vi "SDCP SMF Receiver and Trasmitter - Live Plot.vi"() -> ()   [LabVIEW 2020]
uses:
  Typedefs/SDCP - Standard Message Frame Parameters - FGV - commands.ctl
  Typedefs/SDCP - Serial Port Control - Commands.ctl
  Global Stop.vi
panel:
  in  "SYNC":bool
  out "Update to loop":bool
  out "Ranges to loop":T1(array[cluster])
  out "All offsets":dbl[](array[numeric])
  in  "Offset (%)":dbl
  out "Ranges":T1(array[cluster])
  in  "Set range":bool
  in  "Get range":bool
  in  "Auto range":bool
  in  "Maximum":dbl
  in  "Minimum":dbl
  out "Active Plot Names":string[](array[string])
  out "Value":dbl
  out "Time (ms)":dbl
  in  "Current Parameter":string(combo)
  out "Instantaeneous data":T2(array[cluster])
  in  "Time span (ms)":dbl=20000.0
  in  "Channel 8 enable":bool
  in  "Channel 7 enable":bool
  in  "Channel 6 enable":bool
  in  "Channel 5 enable":bool
  in  "Channel 4 enable":bool
  in  "Channel 3 enable":bool
  in  "Channel 2 enable":bool
  in  "Channel 1 enable":bool
  in  "Channel 8 parameter":string(combo)
  in  "Channel 7 parameter":string(combo)
  in  "Channel 6 parameter":string(combo)
  in  "Channel 5 parameter":string(combo)
  in  "Channel 4 parameter":string(combo)
  in  "Channel 3 parameter":string(combo)
  in  "Channel 2 parameter":string(combo)
  in  "Channel 1 parameter":string(combo)
  in  "Plot file path":path
  out "Live Plot":T3(graph)
  out "Time (ms)":u32
  in  "Stop Application":bool
  in  "Trace file path":path
  in  "Baud rate":u32=9600
  in  "COM Port":refnum<visa-resource-name>
  in  "Parameter file path":path=path "E:/Projects/System Diagnostics and Control Protocol/SDCP_LabVIEW/Parameter Files/Motion_Processing.param"
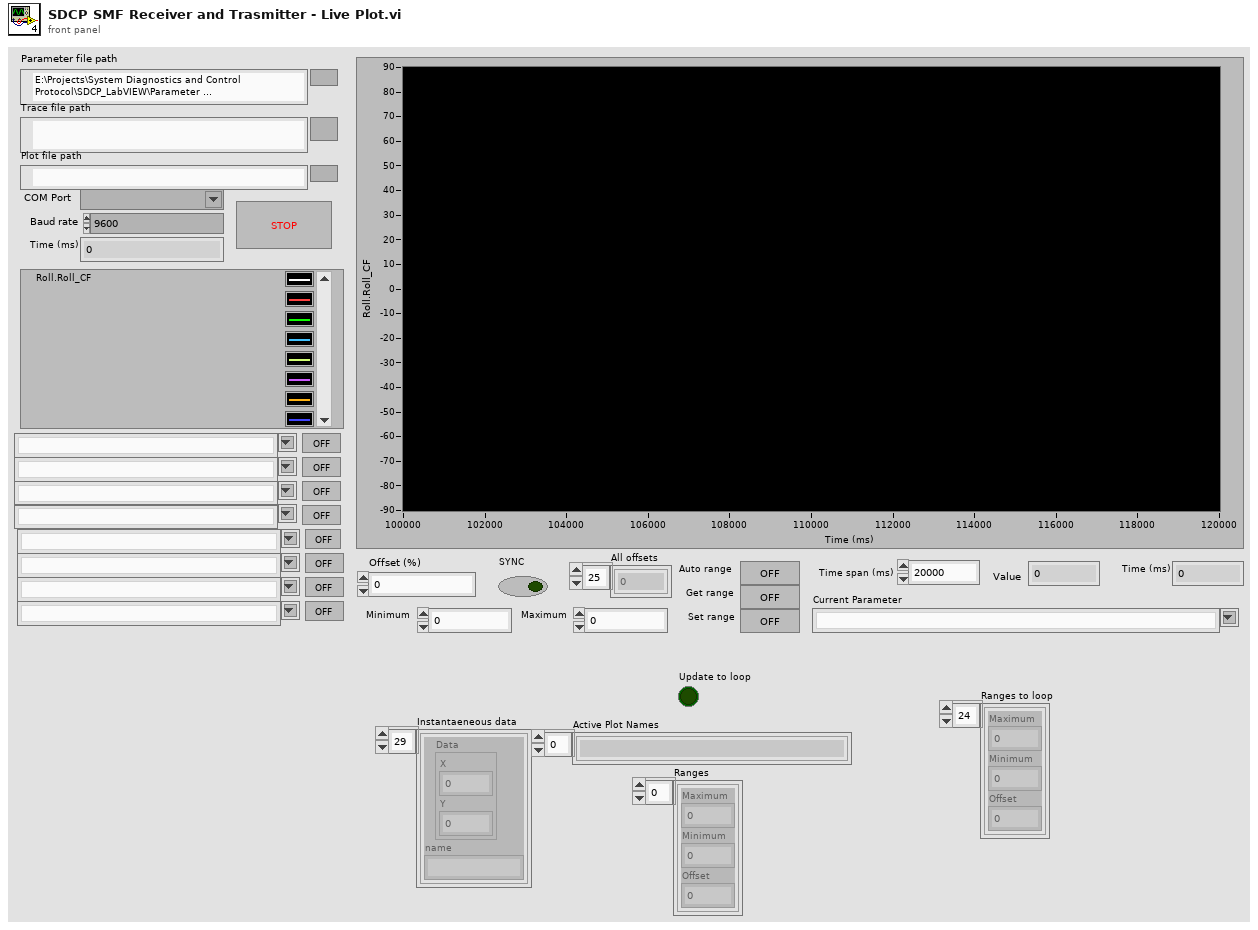
[diagram p1: front panel]
types:
  T1 = cluster{"Maximum":dbl, "Minimum":dbl, "Offset":dbl}[]
  T2 = cluster{"Data":cluster{"X":dbl, "Y":dbl}, "name":string}[]
  T3 = cluster{"Plot data":cluster{"X":dbl, "Y":dbl}[]}[]
  T4 = cluster{"Maximum":dbl, "Minimum":dbl, "Offset":dbl}
  T5 = typedef "SDCP - Serial Port Control - Commands.ctl" = enum16{"Open", "Read", "Write", "Get instance", "Close"}
  T6 = cluster{"data bytes":u8[], "Time (ms)":u32, "Direction":string}
  T7 = typedef "SDCP - Standard Message Frame Parameters - FGV - commands.ctl" = enum16{"Write descriptors", "Read descriptors", "Read values", "Load parameters from file", "Write values", "Read all descriptors"}
  T8 = typedef "SDCP - SMF parameter descriptors.ctl" = cluster{"Frame name":string, "Frame ID":i32, "Data type":string, "Start Position":i32, "Length":i32, "Factor":dbl, "Offset":dbl, "Parameter name":string, "Value":string}
  T9 = cluster{"name":string, "Data":cluster{"X":dbl, "Y":dbl}[]}
  T10 = cluster{"name":string, "Data":cluster{"X":dbl, "Y":dbl}[]}[]
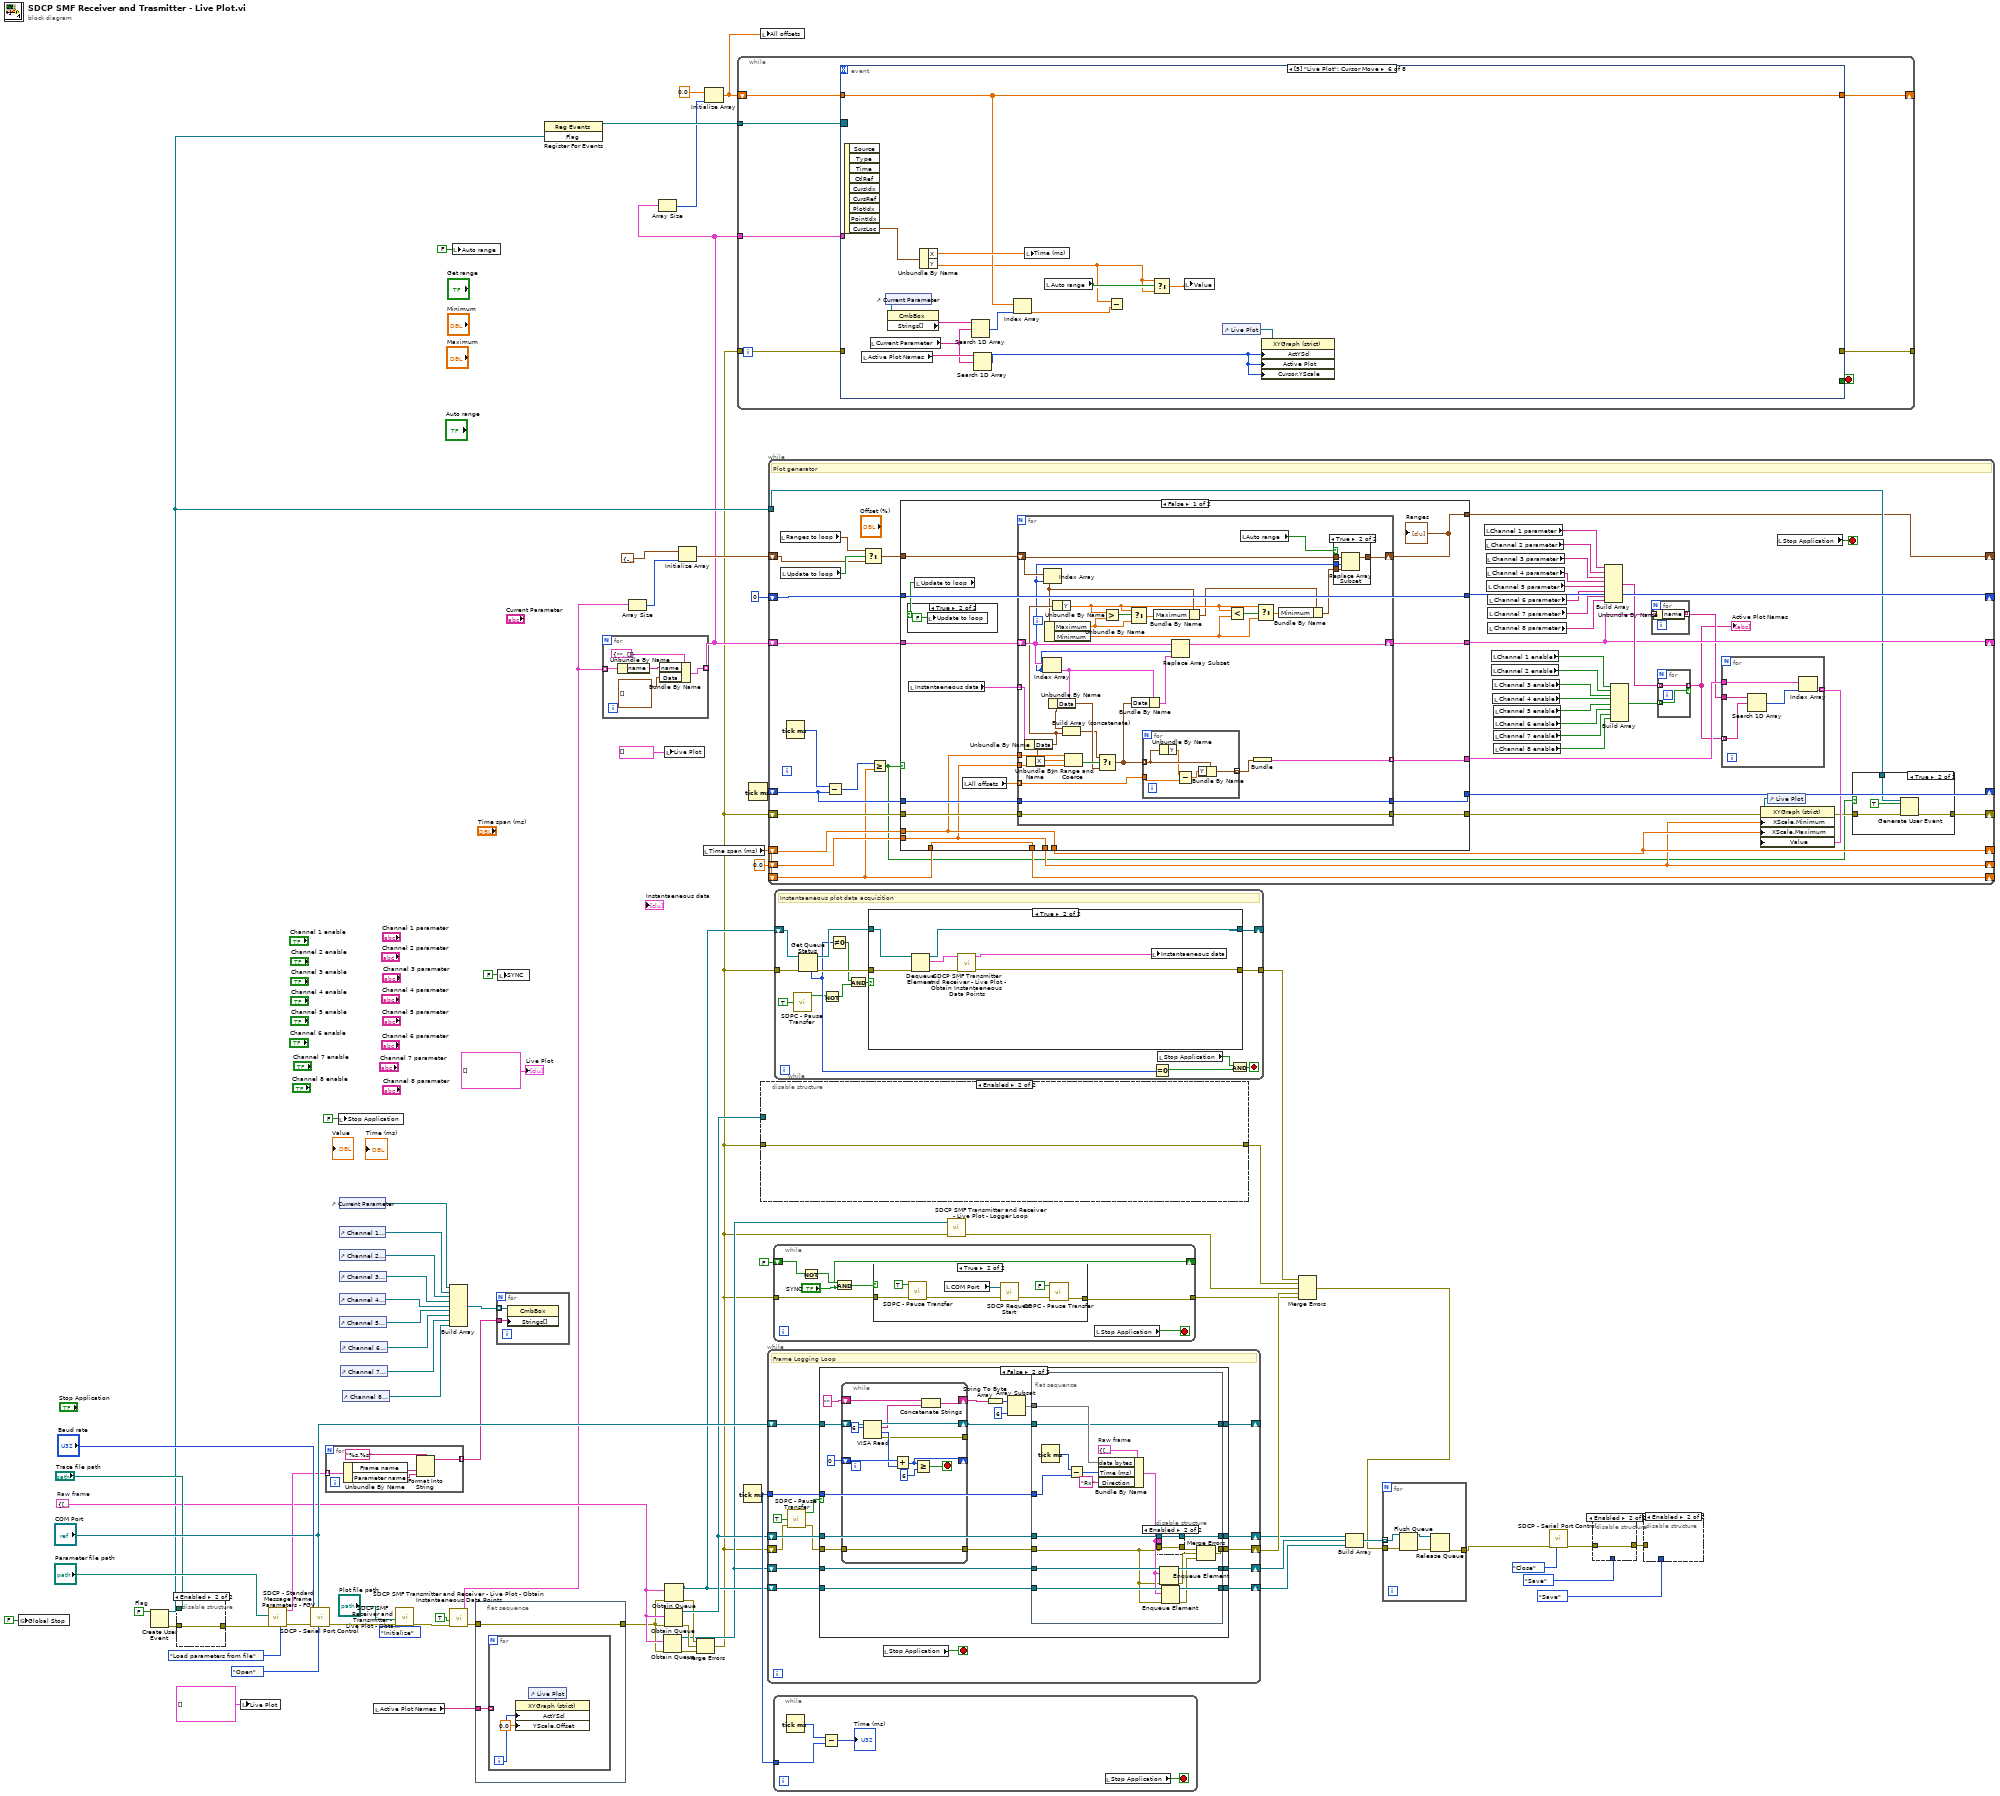
[diagram p0: block diagram]
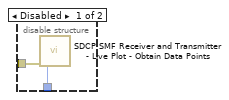
[diagram p3: hidden frame]
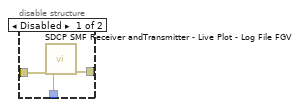
[diagram p4: hidden frame]
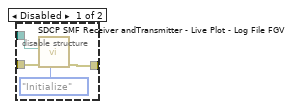
[diagram p5: hidden frame]
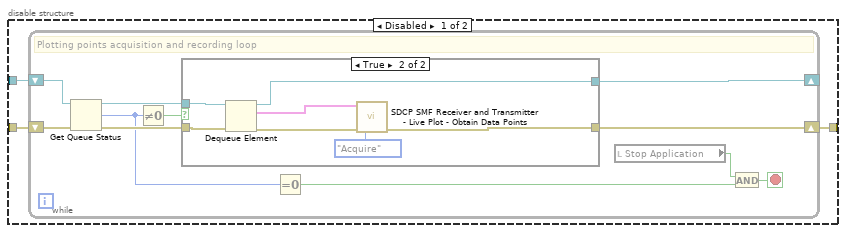
[diagram p6: hidden frame]
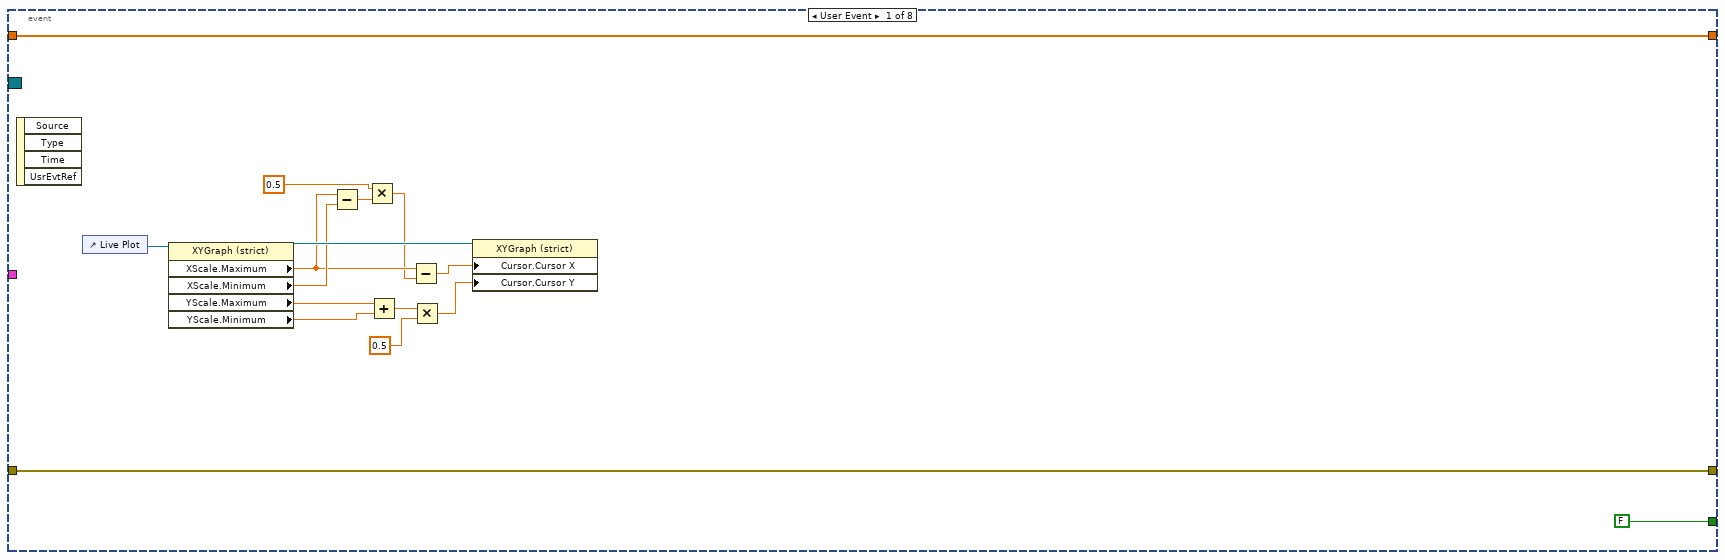
[diagram p8: hidden frame]
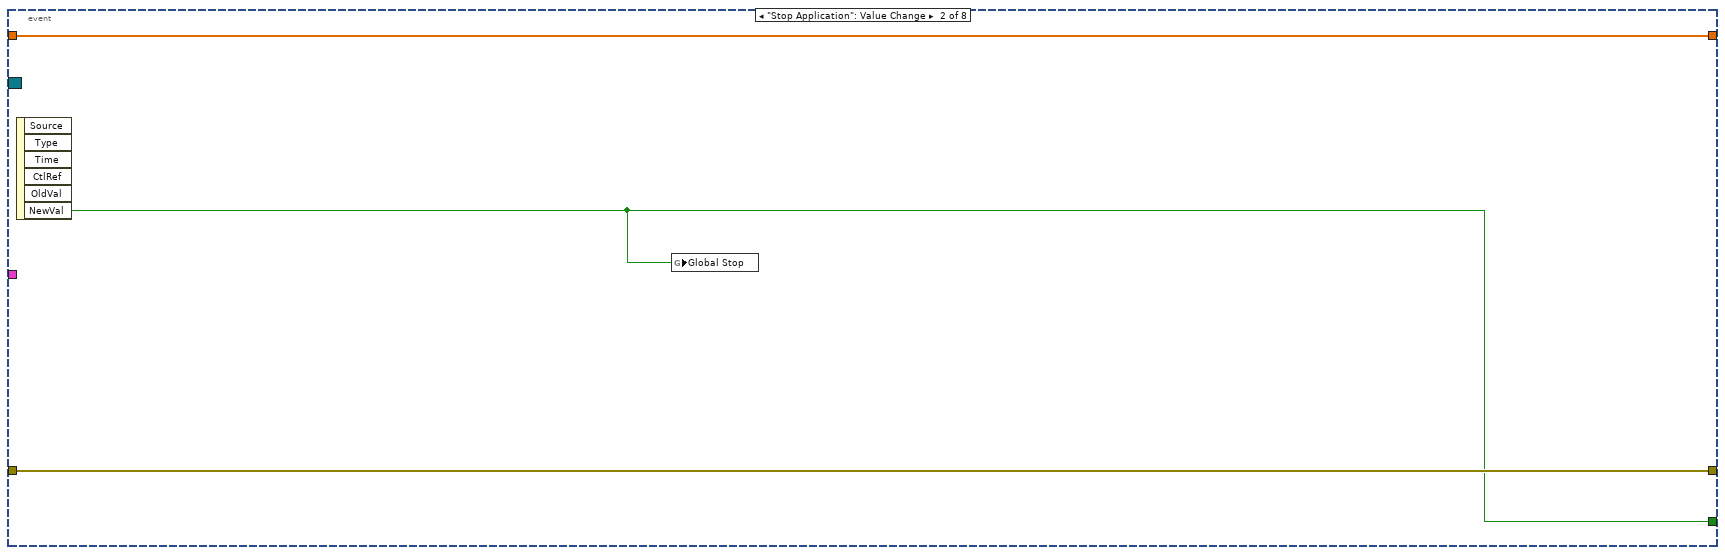
[diagram p9: hidden frame]
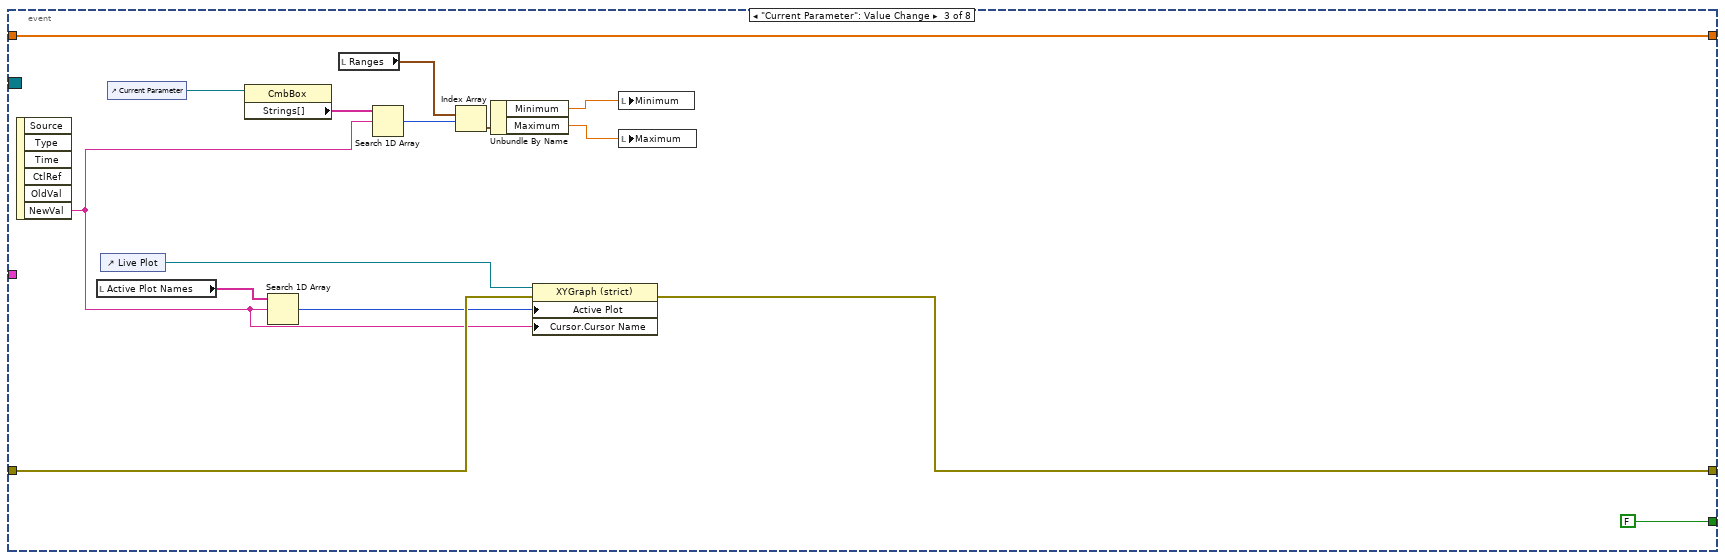
[diagram p10: hidden frame]
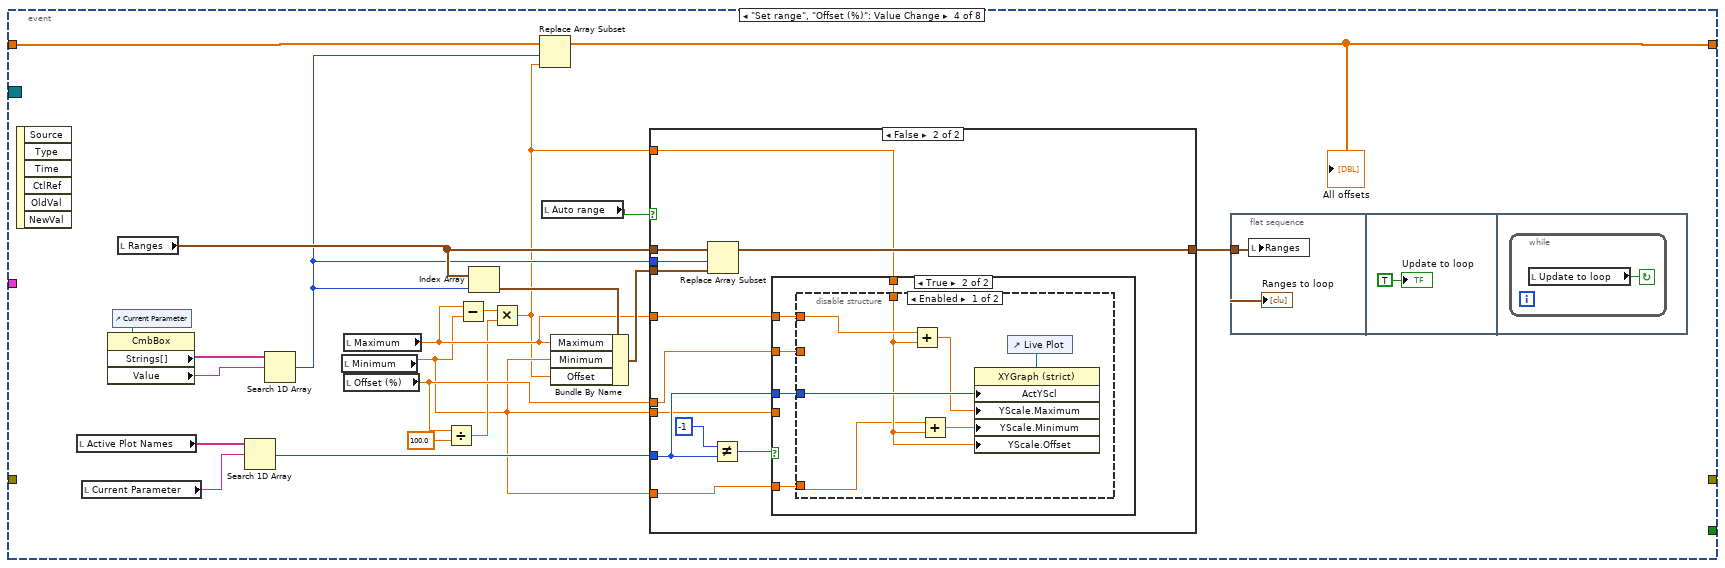
[diagram p11: hidden frame]
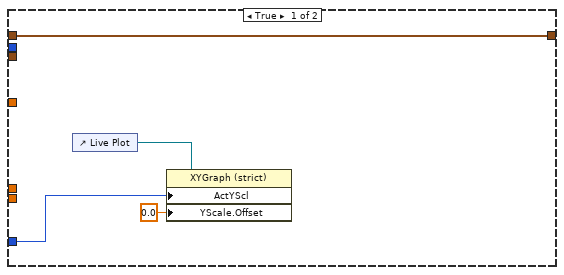
[diagram p12: hidden frame]
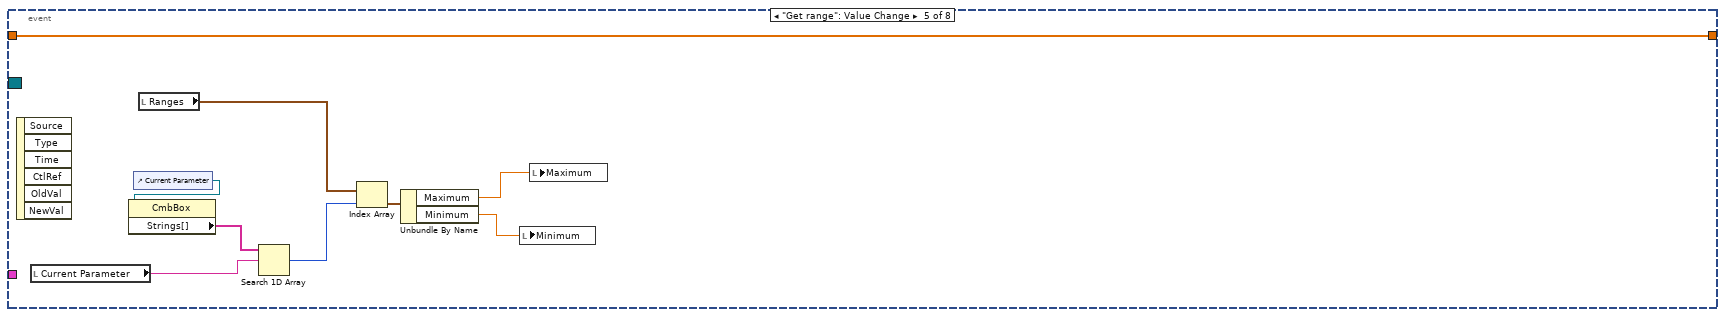
[diagram p15: hidden frame]
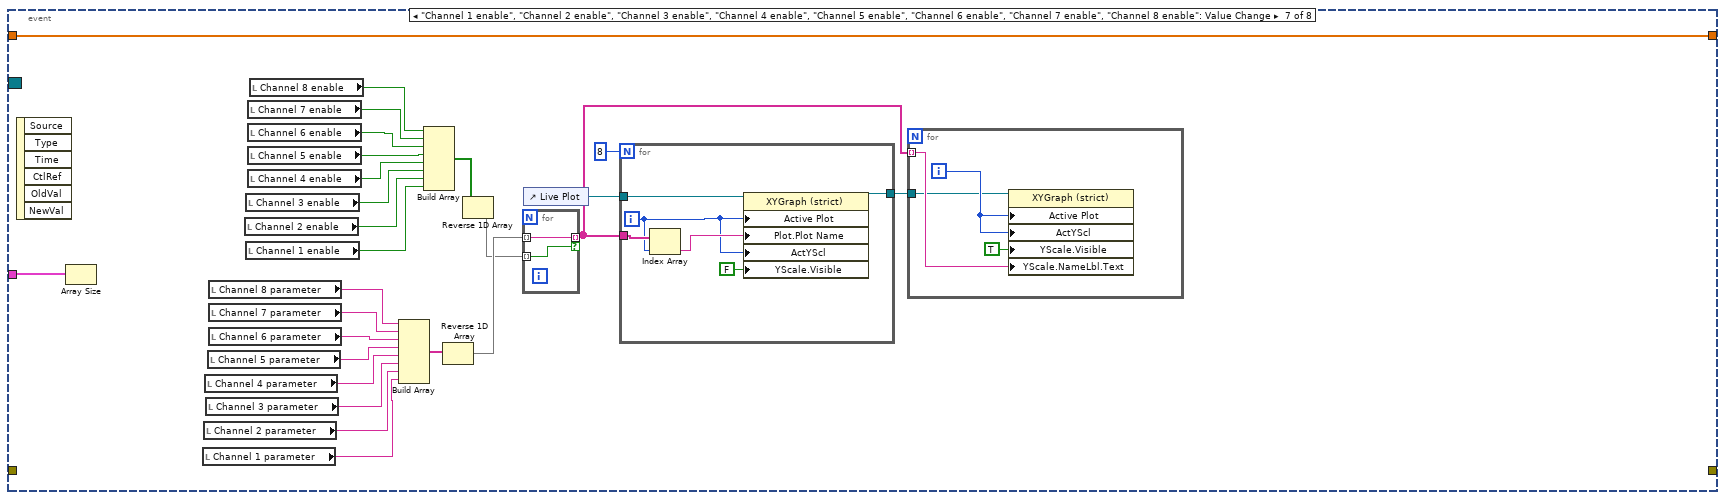
[diagram p16: hidden frame]
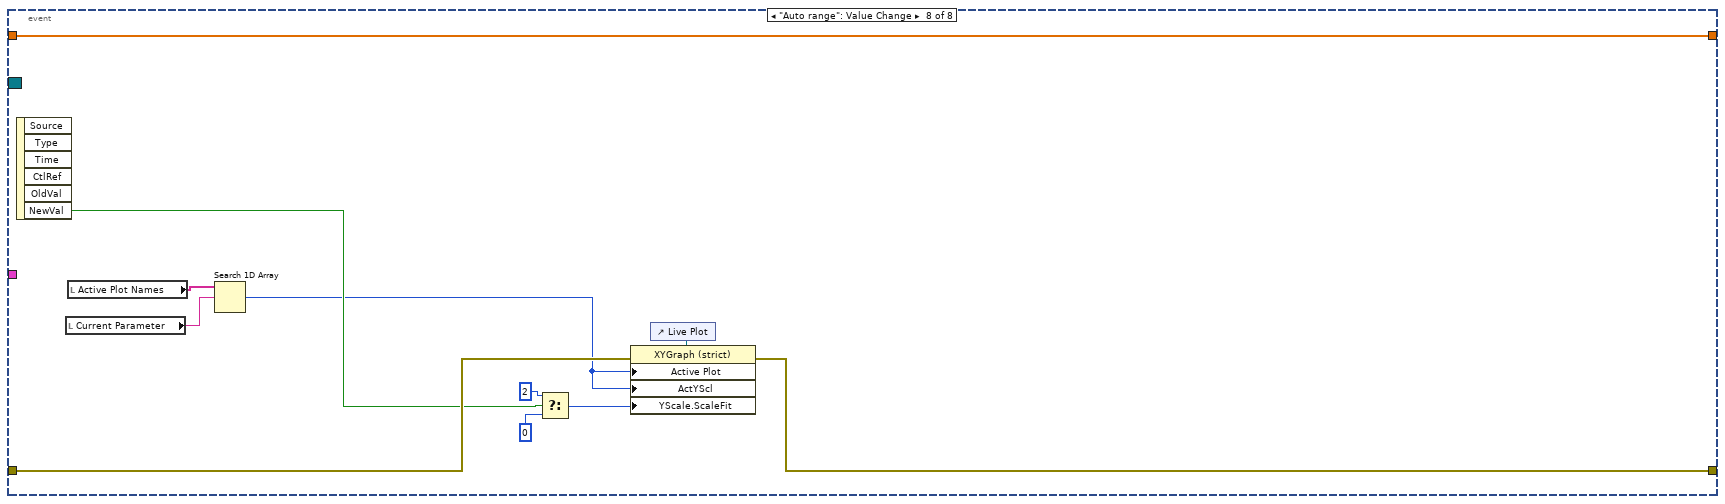
[diagram p17: hidden frame]
diagram:
  w23 = FALSE  # Flag
  w44 = T6 {"data bytes"=[], "Time (ms)"=0, "Direction"=""}  # Raw frame
  n1 = global write "Global Stop.vi" "Global Stop"(FALSE ("Global Stop")) -> ()
  n2 = Create User Event(user event datatype=w23) -> (user event=w21:refnum<user-event>, error out=w24:errorcluster)  [unwired: 1 in]
  n3 = disable-structure shown="Enabled" {
    disable-tunnel: "Trace file path" -> [w81 _]
    disable-tunnel: [w79 w82] -> w62
    disable-tunnel: w24 -> [w78 w82]
    frame Disabled {
      n4 = call "SDCP SMF Receiver andTransmitter - Live Plot - Log File FGV.vi"("error in (no error)"=w78, "Command"=enum16{"Initialize", "Acquire", "Save"}."Initialize", "Trace file path"=w81) -> ("error out"=w79:errorcluster)  [unwired: 4 in]
    }
    frame Enabled {
    }
  }
  n5 = local write "Live Plot"(T3 [] ("Live Plot")) -> ()
  n6 = call "SDCP - Standard Message Frame Parameters - FGV.vi"("Parameter file path"="Parameter file path", "error in (no error)"=w62, "Command"=SDCP_-_Standard_Message_Frame_Parameters_-_FGV_-_commands."Load parameters from file") -> ("SMF Parameters descriptors out"=w57:T8[], "error out"=w75:errorcluster)  [unwired: 4 in]
  n7 = call "SDCP - Serial Port Control.vi"("Command"=SDCP_-_Serial_Port_Control_-_Commands."Open", "VISA resource name"="COM Port", "error in (no error)"=w75, "Baud rate"="Baud rate") -> ("error out"=w46:errorcluster)  [unwired: 4 in, 3 out]
  n8 = for {
    tunnel: w57 -> [w87] mode=indexing
    tunnel: [w83] -> w47 mode=indexing
    n9 = Unbundle By Name(w87) -> ("Frame name"=w85:string, "Parameter name"=w84:string)
    n10 = Format Into String(format string="%s.%s", w85, w84) -> (resulting string=w83:string)  [unwired: 2 in, 1 out]
  }
  n11 = local write "Stop Application"(FALSE ("Stop Application")) -> ()
  n12 = control-ref of="Current Parameter"() -> (w25:refnum<vi>)
  n13 = control-ref of="Channel 1 parameter"() -> (w56:refnum<vi>)
  n14 = control-ref of="Channel 2 parameter"() -> (w55:refnum<vi>)
  n15 = control-ref of="Channel 4 parameter"() -> (w53:refnum<vi>)
  n16 = control-ref of="Channel 3 parameter"() -> (w54:refnum<vi>)
  n17 = control-ref of="Channel 5 parameter"() -> (w52:refnum<vi>)
  n18 = control-ref of="Channel 6 parameter"() -> (w51:refnum<vi>)
  n19 = control-ref of="Channel 7 parameter"() -> (w50:refnum<vi>)
  n20 = control-ref of="Channel 8 parameter"() -> (w49:refnum<vi>)
  n21 = local read "Active Plot Names"() -> (w9:string[])
  n22 = call "SDCP SMF Receiver and Transmitter - Live Plot - Obtain Data Points.vi"("error in (no error)"=w46, "Plot file path"="Plot file path", "Command"=enum16{"Initialize", "Acquire", "Save"}."Initialize") -> ("error out"=w33:errorcluster)  [unwired: 4 in]
  n23 = Build Array(w25, w56, w55, w54, w53, w52, w51, w50, w49) -> (w48:refnum<vi>[])
  n24 = call "SDCP SMF Transmitter and Receiver - Live Plot - Obtain Instantaeneous Data Points.vi"("Initialize ?"=TRUE, "error in (no error)"=w33) -> ("Instantaeneous data"=w19:T2, "error out"=w11:errorcluster)  [unwired: 4 in]
  n25 = local write "Auto range"(FALSE ("Auto range")) -> ()
  n26 = flat-sequence {
    tunnel: w11 -> [w89]
    tunnel: [w89] -> w10
    tunnel: w9 -> [w88]
    frame #0 {
      n27 = for {
        tunnel: w88 -> [_] mode=indexing
        i -> [w91]
        n28 = control-ref of="Live Plot"() -> (w92:refnum<vi>)
        n29 = property class="XYGraph (strict)"(reference=w92, "ActYScl"=w91, "YScale.Offset"=0.0 ("Y Scale.Offset and Multiplier:Offset")) -> ()  [unwired: 1 in, 2 out]
      }
    }
  }
  n30 = for {
    tunnel: w48 -> [w94] mode=indexing
    tunnel: w47 -> [w93]
    n31 = property class="CmbBox"(reference=w94, "Strings[]"=w93) -> ()  [unwired: 1 in, 2 out]
  }
  n32 = local write "SYNC"(FALSE ("SYNC")) -> ()
  n33 = register-events(w21) -> (reference out=w22:refnum<event-registration>)  [unwired: 2 in, 1 out]
  n34 = for {
    tunnel: w19 -> [w99] mode=indexing
    tunnel: [w96] -> w14 mode=indexing
    n35 = Unbundle By Name(w99) -> ("name"=w97:string)
    n36 = Bundle By Name(cluster=T9 {"name"="", "Data"=[]}, "name"=w97, "Data"=cluster{"X":dbl, "Y":dbl}[] []) -> (w96:T9)
  }
  n37 = Array Size(array=w19) -> (size(s)=w18:i32)
  n38 = Array Size(array=w14) -> (size(s)=w13:i32)
  n39 = Obtain Queue(element data type=w44, error in (no error)=w10) -> (queue out=w7:refnum<queue>, error out=w70:errorcluster)  [unwired: 3 in, 1 out]
  n40 = local write "Live Plot"(cluster{"Data":cluster{"X":dbl, "Y":dbl}[]}[] []) -> ()
  n41 = Obtain Queue(element data type=w44, error in (no error)=w10) -> (queue out=w63:refnum<queue>, error out=w71:errorcluster)  [unwired: 3 in, 1 out]
  n42 = Obtain Queue(element data type=w44, error in (no error)=w10) -> (queue out=w35:refnum<queue>, error out=w43:errorcluster)  [unwired: 3 in, 1 out]
  n43 = Initialize Array(T4 {"Maximum"=-1000000000.0, "Minimum"=1000000000.0, "Offset"=0.0}, w18) -> (w17:T1)
  n44 = Merge Errors(w43, w71, w70) -> (w4:errorcluster)
  n45 = local read "Time span (ms)"() -> (w26:dbl)
  n46 = Initialize Array(0.0, w13) -> (w12:dbl[])
  n47 = while {
    tunnel: w4 -> [w106]
    tunnel: [w105] -> _
    tunnel: w22 -> [w103]
    tunnel: w14 -> [w102]
    shift-right: [w100] -> _
    shift-left: w12 -> [w101]
    stop <- w104 stop-if-true
    n48 = event shown="[5] \"Live Plot\": Cursor Move" {
      selector: w103 -> [_ _ _ _ _ _ _ _]
      dyn-events: _ -> [_ _ _ _ _ _ _ _]
      timeout: _ -> [_ _ _ _ _ _ _ _]
      tunnel: w106 -> [w122 w125 w139 _ _ _ _ w264]
      tunnel: [w122 w125 w136 _ _ _ _ w263] -> w105
      tunnel: [FALSE w123 FALSE ("NewVal") _ _ _ _ _] -> w104
      tunnel: w102 -> [_ _ _ _ _ _ w225 _]
      tunnel: w101 -> [w107 w124 w127 w146 w193 w206 w216 w254]
      tunnel: [w107 w124 w127 w144 w193 w206 w216 w254] -> w100
      event User Event {
        n49 = event-data() -> ()  [unwired: 1 in, 4 out]
        n50 = control-ref of="Live Plot"() -> (w120:refnum<vi>)
        n51 = property class="XYGraph (strict)"(reference=w120) -> (reference out=w115:refnum<vi>, "XScale.Maximum"=w112:dbl, "XScale.Minimum"=w113:dbl, "YScale.Maximum"=w119:dbl, "YScale.Minimum"=w118:dbl)  [unwired: 1 in, 1 out]
        n52 = Subtract(x=w112, y=w113) -> (x-y=w111:dbl)
        n53 = Multiply(x=0.5, y=w111) -> (x*y=w109:dbl)
        n54 = Add(x=w119, y=w118) -> (x+y=w117:dbl)
        n55 = Subtract(x=w112, y=w109) -> (x-y=w108:dbl)
        n56 = Multiply(x=w117, y=0.5) -> (x*y=w114:dbl)
        n57 = property class="XYGraph (strict)"(reference=w115, "Cursor.Cursor X"=w108, "Cursor.Cursor Y"=w114) -> ()  [unwired: 1 in, 2 out]
      }
      event "Stop Application": Value Change {
        n58 = event-data() -> ("NewVal"=w123:bool)  [unwired: 1 in, 5 out]
        n59 = global write "Global Stop.vi" "Global Stop"(w123) -> ()
      }
      event "Current Parameter": Value Change {
        n60 = event-data() -> ("NewVal"=w126:string)  [unwired: 1 in, 5 out]
        n61 = local read "Active Plot Names"() -> (w135:string[])
        n62 = control-ref of="Live Plot"() -> (w138:refnum<vi>)
        n63 = control-ref of="Current Parameter"() -> (w134:refnum<vi>)
        n64 = property class="CmbBox"(reference=w134) -> ("Strings[]"=w133:string[])  [unwired: 1 in, 2 out]
        n65 = Search 1D Array(1D array=w135, element=w126) -> (index of element=w137:i32)  [unwired: 1 in]
        n66 = local read "Ranges"() -> (w132:T1)
        n67 = Search 1D Array(1D array=w133, element=w126) -> (index of element=w131:i32)  [unwired: 1 in]
        n68 = Index Array(array=w132, index=w131) -> (element=w130:T4)
        n69 = Unbundle By Name(w130) -> ("Minimum"=w129:dbl, "Maximum"=w128:dbl)
        n70 = property class="XYGraph (strict)"(reference=w138, error in=w139, "Active Plot"=w137, "Cursor.Cursor Name"=w126) -> (error out=w136:errorcluster)  [unwired: 1 out]
        n71 = local write "Minimum"(w129) -> ()
        n72 = local write "Maximum"(w128) -> ()
      }
      event "Set range", "Offset (%)": Value Change {
        n73 = event-data() -> ()  [unwired: 1 in, 6 out]
        n74 = local read "Active Plot Names"() -> (w154:string[])
        n75 = local read "Current Parameter"() -> (w153:string)
        n76 = control-ref of="Current Parameter"() -> (w161:refnum<vi>)
        n77 = property class="CmbBox"(reference=w161) -> ("Strings[]"=w160:string[], "Value"=w159:string)  [unwired: 1 in, 2 out]
        n78 = local read "Ranges"() -> (w158:T1)
        n79 = Search 1D Array(1D array=w154, element=w153) -> (index of element=w152:i32)  [unwired: 1 in]
        n80 = Search 1D Array(1D array=w160, element=w159) -> (index of element=w145:i32)  [unwired: 1 in]
        n81 = local read "Minimum"() -> (w143:dbl)
        n82 = local read "Maximum"() -> (w151:dbl)
        n83 = local read "Offset (%)"() -> (w149:dbl)
        n84 = Divide(x=w149, y=100.0) -> (x/y=w147:dbl)
        n85 = Subtract(x=w151, y=w143) -> (x-y=w150:dbl)
        n86 = Index Array(array=w158, index=w145) -> (element=w157:T4)
        n87 = Multiply(x=w150, y=w147) -> (x*y=w142:dbl)
        n88 = Replace Array Subset(array=w146, new element=w142, index=w145) -> (w144:dbl[])
        "All offsets" <- w144
        n89 = local read "Auto range"() -> (w155:bool)
        n90 = Bundle By Name(cluster=w157, "Maximum"=w151, "Minimum"=w143, "Offset"=w142) -> (w156:T4)
        n91 = case shown="False" w155 {
          tunnel: w158 -> [w168 w180]
          tunnel: w145 -> [_ w179]
          tunnel: w156 -> [_ w178]
          tunnel: [w168 w177] -> w141
          tunnel: w152 -> [w166 w174]
          tunnel: w151 -> [_ w173]
          tunnel: w143 -> [_ w172]
          tunnel: w149 -> [_ w171]
          tunnel: w143 -> [_ w170]
          tunnel: w142 -> [_ w169]
          frame True {
            n92 = control-ref of="Live Plot"() -> (w167:refnum<vi>)
            n93 = property class="XYGraph (strict)"(reference=w167, "ActYScl"=w166, "YScale.Offset"=0.0 ("Y Scale.Offset and Multiplier:Offset")) -> ()  [unwired: 1 in, 2 out]
          }
          frame False {
            n94 = Replace Array Subset(array=w180, new element=w178, index=w179) -> (w177:T1)
            n95 = Not Equal?(x=-1, y=w174) -> (x != y?=w175:bool)
            n96 = case shown="True" w175 {
              tunnel: w174 -> [_ w185]
              tunnel: w173 -> [_ w184]
              tunnel: w172 -> [_ _]
              tunnel: w171 -> [_ w183]
              tunnel: w170 -> [_ w182]
              tunnel: w169 -> [_ w181]
              frame False {
              }
              frame True {
                n97 = disable-structure shown="Enabled" {
                  disable-tunnel: w185 -> [w191 _]
                  disable-tunnel: w184 -> [w188 _]
                  disable-tunnel: w183 -> [_ _]
                  disable-tunnel: w182 -> [w186 _]
                  disable-tunnel: w181 -> [w187 _]
                  frame Enabled {
                    n98 = Add(x=w188, y=w187) -> (x+y=w190:dbl)
                    n99 = Add(x=w186, y=w187) -> (x+y=w189:dbl)
                    n100 = control-ref of="Live Plot"() -> (w192:refnum<vi>)
                    n101 = property class="XYGraph (strict)"(reference=w192, "ActYScl"=w191, "YScale.Maximum"=w190, "YScale.Minimum"=w189, "YScale.Offset"=w187) -> ()  [unwired: 1 in, 2 out]
                  }
                  frame Disabled {
                  }
                }
              }
            }
          }
        }
        n102 = flat-sequence {
          tunnel: w141 -> [w162]
          frame #0 {
            n103 = local write "Ranges"(w162) -> ()
            "Ranges to loop" <- w162
          }
          frame #1 {
            "Update to loop" <- TRUE ("Update to loop")
          }
          frame #2 {
            n104 = while {
              stop <- w164 continue-if-true
              n105 = local read "Update to loop"() -> (w164:bool)
            }
          }
        }
      }
      event "Get range": Value Change {
        n106 = event-data() -> ()  [unwired: 1 in, 6 out]
        n107 = local read "Current Parameter"() -> (w199:string)
        n108 = control-ref of="Current Parameter"() -> (w201:refnum<vi>)
        n109 = property class="CmbBox"(reference=w201) -> ("Strings[]"=w200:string[])  [unwired: 1 in, 2 out]
        n110 = local read "Ranges"() -> (w198:T1)
        n111 = Search 1D Array(1D array=w200, element=w199) -> (index of element=w197:i32)  [unwired: 1 in]
        n112 = Index Array(array=w198, index=w197) -> (element=w196:T4)
        n113 = Unbundle By Name(w196) -> ("Maximum"=w195:dbl, "Minimum"=w194:dbl)
        n114 = local write "Minimum"(w194) -> ()
        n115 = local write "Maximum"(w195) -> ()
      }
      event "Live Plot": Cursor Move {
        n116 = event-data() -> ("CursLoc"=w215:cluster{"X":dbl, "Y":dbl})  [unwired: 1 in, 8 out]
        n117 = local read "Active Plot Names"() -> (w209:string[])
        n118 = local read "Current Parameter"() -> (w208:string)
        n119 = control-ref of="Current Parameter"() -> (w213:refnum<vi>)
        n120 = property class="CmbBox"(reference=w213) -> ("Strings[]"=w212:string[])  [unwired: 1 in, 2 out]
        n121 = Unbundle By Name(w215) -> ("X"=w214:dbl, "Y"=w202:dbl)
        n122 = Search 1D Array(1D array=w212, element=w208) -> (index of element=w205:i32)  [unwired: 1 in]
        n123 = Search 1D Array(1D array=w209, element=w208) -> (index of element=w203:i32)  [unwired: 1 in]
        n124 = Index Array(array=w206, index=w205) -> (element=w204:dbl)
        n125 = local write "Time (ms)"(w214) -> ()
        n126 = local read "Auto range"() -> (w211:bool)
        n127 = Subtract(x=w202, y=w204) -> ()  [unwired: 1 out]
        n128 = Select(t=w202, s=w211, f=w202) -> (s? t:f=w210:dbl)
        n129 = local write "Value"(w210) -> ()
        n130 = control-ref of="Live Plot"() -> (w207:refnum<vi>)
        n131 = property class="XYGraph (strict)"(reference=w207, "ActYScl"=w203, "Active Plot"=w203, "Cursor.YScale"=w203) -> ()  [unwired: 1 in, 2 out]
      }
      event "Channel 1 enable", "Channel 2 enable", "Channel 3 enable", "Channel 4 enable", "Channel 5 enable", "Channel 6 enable", "Channel 7 enable", "Channel 8 enable": Value Change {
        n132 = event-data() -> ()  [unwired: 1 in, 6 out]
        n133 = Array Size(array=w225) -> ()  [unwired: 1 out]
        n134 = local read "Channel 1 parameter"() -> (w226:string)
        n135 = local read "Channel 2 parameter"() -> (w227:string)
        n136 = local read "Channel 4 parameter"() -> (w229:string)
        n137 = local read "Channel 3 parameter"() -> (w228:string)
        n138 = local read "Channel 5 parameter"() -> (w230:string)
        n139 = local read "Channel 8 parameter"() -> (w233:string)
        n140 = local read "Channel 7 parameter"() -> (w232:string)
        n141 = local read "Channel 6 parameter"() -> (w231:string)
        n142 = local read "Channel 2 enable"() -> (w235:bool)
        n143 = local read "Channel 3 enable"() -> (w236:bool)
        n144 = local read "Channel 1 enable"() -> (w234:bool)
        n145 = local read "Channel 7 enable"() -> (w240:bool)
        n146 = local read "Channel 6 enable"() -> (w239:bool)
        n147 = local read "Channel 5 enable"() -> (w238:bool)
        n148 = local read "Channel 4 enable"() -> (w237:bool)
        n149 = local read "Channel 8 enable"() -> (w241:bool)
        n150 = Build Array(w233, w232, w231, w230, w229, w228, w227, w226) -> (w223:string[])
        n151 = Build Array(w241, w240, w239, w238, w237, w236, w235, w234) -> (w222:bool[])
        n152 = Reverse 1D Array(array=w223) -> (reversed array=w220:string[])
        n153 = Reverse 1D Array(array=w222) -> (reversed array=w219:bool[])
        n154 = for {
          tunnel: w220 -> [w253] mode=indexing
          tunnel: w219 -> [w252] mode=indexing
          tunnel: [w253] -> w218 mode=indexing if=w252
        }
        n155 = control-ref of="Live Plot"() -> (w221:refnum<vi>)
        n156 = for {
          N: 8 -> [_]
          tunnel: w221 -> [w251]
          tunnel: w218 -> [w250]
          tunnel: [w248] -> w217
          i -> [w247]
          n157 = Index Array(array=w250, index=w247) -> (element=w249:string)
          n158 = property class="XYGraph (strict)"(reference=w251, "Active Plot"=w247, "Plot.Plot Name"=w249, "ActYScl"=w247, "YScale.Visible"=FALSE ("Y Scale.Visible")) -> (reference out=w248:refnum<vi>)  [unwired: 1 in, 1 out]
        }
        n159 = for {
          tunnel: w218 -> [w244] mode=indexing
          tunnel: w217 -> [w242]
          i -> [w245]
          n160 = property class="XYGraph (strict)"(reference=w242, "Active Plot"=w245, "ActYScl"=w245, "YScale.Visible"=TRUE ("Y Scale.Visible"), "YScale.NameLbl.Text"=w244) -> ()  [unwired: 1 in, 2 out]
        }
      }
      event "Auto range": Value Change {
        n161 = event-data() -> ("NewVal"=w258:bool)  [unwired: 1 in, 5 out]
        n162 = local read "Current Parameter"() -> (w256:string)
        n163 = local read "Active Plot Names"() -> (w257:string[])
        n164 = Search 1D Array(1D array=w257, element=w256) -> (index of element=w255:i32)  [unwired: 1 in]
        n165 = Select(t=2, s=w258, f=0) -> (s? t:f=w259:i32)
        n166 = control-ref of="Live Plot"() -> (w262:refnum<vi>)
        n167 = property class="XYGraph (strict)"(reference=w262, error in=w264, "Active Plot"=w255, "ActYScl"=w255, "YScale.ScaleFit"=w259) -> (error out=w263:errorcluster)  [unwired: 1 out]
      }
    }
  }
  n168 = Tick Count (ms)() -> (millisecond timer value=w64:u32)
  n169 = Tick Count (ms)() -> (millisecond timer value=w31:u32)
  n170 = local write "All offsets"(w12) -> ()
  n171 = disable-structure shown="Enabled" {
    disable-tunnel: w63 -> [w267 _]
    disable-tunnel: [w266 w288] -> w42
    disable-tunnel: w4 -> [w265 w288]
    frame Disabled {
      n172 = while {
        shift-right: [w272] -> _
        shift-left: w267 -> [w277]
        shift-right: [w274] -> w266
        shift-left: w265 -> [w278]
        stop <- w270 stop-if-true
        # "Plotting points acquisition and recording loop"
        n173 = Get Queue Status(queue=w277, error in (no error)=w278) -> (queue out=w273:refnum<queue>, error out=w275:errorcluster, # elements in queue=w271:i32)  [unwired: 1 in, 5 out]
        n174 = Not Equal To 0?(x=w271) -> (x != 0?=w276:bool)
        n175 = case shown="True" w276 {
          tunnel: w275 -> [w280 w287]
          tunnel: [w280 w282] -> w274
          tunnel: w273 -> [w279 w286]
          tunnel: [w279 w285] -> w272
          frame False {
          }
          frame True {
            n176 = Dequeue Element(queue=w286, error in (no error)=w287) -> (queue out=w285:refnum<queue>, element=w283:T6, error out=w284:errorcluster)  [unwired: 1 in, 1 out]
            n177 = call "SDCP SMF Receiver and Transmitter - Live Plot - Obtain Data Points.vi"("error in (no error)"=w284, "Command"=enum16{"Initialize", "Acquire", "Save"}."Acquire", "Raw frame"=w283) -> ("error out"=w282:errorcluster)  [unwired: 4 in]
          }
        }
        n178 = Equal To 0?(x=w271) -> (x = 0?=w268:bool)
        n179 = local read "Stop Application"() -> (w269:bool)
        n180 = And(x=w269, y=w268) -> (x .and. y?=w270:bool)
      }
    }
    frame Enabled {
    }
  }
  n181 = while {
    tunnel: w64 -> [w302]
    shift-right: [w300] -> _
    shift-left: "COM Port" -> [w303]
    shift-right: [w301] -> w65
    shift-left: w4 -> [w291]
    shift-right: [w298] -> w41
    shift-left: w63 -> [w299]
    shift-right: [w296] -> w40
    shift-left: w7 -> [w297]
    shift-right: [w293] -> w39
    shift-left: w35 -> [w294]
    stop <- w295 stop-if-true
    # "Frame Logging Loop"
    n182 = call "SDPC - Pause Transfer.vi"("error in (no error)"=w291, "RD/nWR"=TRUE) -> ("error out"=w289:errorcluster, "Transfer paused"=w290:bool)  [unwired: 2 in]
    n183 = case shown="False" w290 {
      tunnel: w303 -> [w308 w327]
      tunnel: w302 -> [_ w320]
      tunnel: [w306 w319] -> w301
      tunnel: [w308 w317] -> w300
      tunnel: w299 -> [w307 w316]
      tunnel: [w307 w315] -> w298
      tunnel: w297 -> [w305 w314]
      tunnel: [w305 w313] -> w296
      tunnel: w294 -> [w304 w312]
      tunnel: [w304 w311] -> w293
      tunnel: w289 -> [w306 w310]
      frame True {
      }
      frame False {
        n184 = while {
          shift-right: [w365] -> w318
          shift-left: w327 -> [w366]
          shift-right: [w357] -> w324
          shift-left: "" -> [w359]
          shift-right: [w361] -> _
          shift-left: 0 -> [w364]
          tunnel: w310 -> [w355]
          tunnel: [w355] -> w309
          tunnel: [w354] -> _
          stop <- w360 stop-if-true
          n185 = VISA Read(VISA resource name=w366, byte count=u32 6) -> (VISA resource name out=w365:refnum<visa-resource-name>, read buffer=w358:string, return count=w363:u32, error out=w354:errorcluster)  [unwired: 1 in]
          n186 = Add(x=w364, y=w363) -> (x+y=w361:u32)
          n187 = Greater Or Equal?(x=w361, y=u32 6) -> (x >= y?=w360:bool)
          n188 = Concatenate Strings(w359, w358) -> (w357:string)
        }
        n189 = String To Byte Array(string=w324) -> (unsigned byte array=w323:u8[])
        n190 = Array Subset(array=w323, length=6) -> (w321:u8[])  [unwired: 1 in]
        n191 = flat-sequence {
          tunnel: w321 -> [w337]
          tunnel: w320 -> [w345]
          tunnel: w309 -> [w332]
          tunnel: [w331] -> w319
          tunnel: w318 -> [w336]
          tunnel: [w336] -> w317
          tunnel: w316 -> [w342]
          tunnel: [w341] -> w315
          tunnel: w314 -> [w340]
          tunnel: [w339] -> w313
          tunnel: w312 -> [w335]
          tunnel: [w333] -> w311
          frame #0 {
            w344 = T6 {"data bytes"=[], "Time (ms)"=0, "Direction"=""}  # Raw frame
            n192 = Tick Count (ms)() -> (millisecond timer value=w346:u32)
            n193 = Subtract(x=w346, y=w345) -> (x-y=w343:u32)
            n194 = Bundle By Name(cluster=w344, "data bytes"=w337, "Time (ms)"=w343, "Direction"="Rx") -> (w334:T6)
            n195 = disable-structure shown="Enabled" {
              disable-tunnel: w342 -> [w351 w352]
              disable-tunnel: [w350 w352] -> w341
              disable-tunnel: w334 -> [w349 _]
              disable-tunnel: w332 -> [w348 w353]
              disable-tunnel: [w347 w353] -> w330
              frame Disabled {
                n196 = Enqueue Element(queue=w351, element=w349, error in (no error)=w348) -> (queue out=w350:refnum<queue>, error out=w347:errorcluster)  [unwired: 1 in, 1 out]
              }
              frame Enabled {
              }
            }
            n197 = Enqueue Element(queue=w340, element=w334, error in (no error)=w332) -> (queue out=w339:refnum<queue>, error out=w329:errorcluster)  [unwired: 1 in, 1 out]
            n198 = Enqueue Element(queue=w335, element=w334, error in (no error)=w332) -> (queue out=w333:refnum<queue>, error out=w328:errorcluster)  [unwired: 1 in, 1 out]
            n199 = Merge Errors(w330, w329, w328) -> (w331:errorcluster)
          }
        }
      }
    }
    n200 = local read "Stop Application"() -> (w295:bool)
  }
  n201 = while {
    shift-right: [w375] -> _
    shift-left: w4 -> [w412]
    shift-right: [w411] -> _
    shift-left: w31 -> [w409]
    shift-right: [w384] -> _
    shift-left: w14 -> [w410]
    shift-right: [w408] -> _
    shift-left: 0 -> [w407]
    shift-right: [w382] -> _
    shift-left: w26 -> [w381]
    shift-right: [w379] -> _
    shift-left: 0.0 -> [w380]
    shift-right: [w378] -> _
    shift-left: w26 -> [w377]
    tunnel: w21 -> [w374]
    shift-right: [w371] -> _
    shift-left: w17 -> [w369]
    stop <- w415 stop-if-true
    # "Plot generator"
    n202 = local read "Ranges to loop"() -> (w367:T1)
    n203 = local read "Update to loop"() -> (w370:bool)
    n204 = Tick Count (ms)() -> (millisecond timer value=w414:u32)
    n205 = Subtract(x=w414, y=w409) -> (x-y=w413:u32)
    n206 = Select(t=w367, s=w370, f=w369) -> (s? t:f=w368:T1)
    n207 = Greater Or Equal?(x=w413, y=w377) -> (x >= y?=w373:bool)
    n208 = case shown="False" w373 {
      tunnel: w412 -> [w440 w506]
      tunnel: [w439 w507] -> w406
      tunnel: [w442 w511] -> w411
      tunnel: w410 -> [w445 w510]
      tunnel: [w441 w508] -> w384
      tunnel: w409 -> [w443 _]
      tunnel: [w437 w505] -> w386
      tunnel: w407 -> [w438 w504]
      tunnel: [w438 w503] -> w408
      tunnel: [w436 w500] -> w382
      tunnel: [w435 w499] -> w379
      tunnel: w381 -> [w436 w502]
      tunnel: w380 -> [w435 w501]
      tunnel: [w434 w497] -> w378
      tunnel: w377 -> [w434 w496]
      tunnel: w368 -> [w433 w490]
      tunnel: [w432 w489] -> w371
      frame False {
        n209 = local read "Instantaeneous data"() -> (w444:T2)
        n210 = local read "Update to loop"() -> (w430:bool)
        n211 = case shown="True" w430 {
          frame False {
          }
          frame True {
            n212 = local write "Update to loop"(FALSE ("Update to loop")) -> ()
          }
        }
        n213 = local read "All offsets"() -> (w431:dbl[])
        n214 = for {
          shift-right: [w474] -> w441
          shift-left: w445 -> [w476]
          tunnel: w444 -> [w477] mode=indexing
          tunnel: w443 -> [w473]
          tunnel: [w473] -> w442
          tunnel: w440 -> [w472]
          tunnel: [w472] -> w439
          tunnel: [w471] -> w437 mode=indexing
          tunnel: w436 -> [w466]
          tunnel: w435 -> [w465]
          shift-right: [w451] -> w432
          shift-left: w433 -> [w454]
          tunnel: w431 -> [w448] mode=indexing
          i -> [w453]
          n215 = Unbundle By Name(w477) -> ("Data"=w464:cluster{"X":dbl, "Y":dbl})
          n216 = Unbundle By Name(w464) -> ("X"=w470:dbl)
          n217 = Index Array(array=w476, index=w453) -> (element=w478:T9)
          n218 = Index Array(array=w454, index=w453) -> (element=w460:T4)
          n219 = Unbundle By Name(w460) -> ("Maximum"=w462:dbl, "Minimum"=w457:dbl)
          n220 = Unbundle By Name(w478) -> ("Data"=w468:cluster{"X":dbl, "Y":dbl}[])
          n221 = Unbundle By Name(w464) -> ("Y"=w458:dbl)
          n222 = Build Array (concatenate)(w468, w464) -> (w467:cluster{"X":dbl, "Y":dbl}[])
          n223 = In Range and Coerce(upper limit=w466, x=w470, lower limit=w465) -> (In Range?=w469:bool)  [unwired: 1 out]
          n224 = Select(t=w467, s=w469, f=w468) -> (s? t:f=w449:cluster{"X":dbl, "Y":dbl}[])
          n225 = Greater?(x=w458, y=w462) -> (0:w463:bool)
          n226 = Select(t=w458, s=w463, f=w462) -> (s? t:f=w461:dbl)
          n227 = Bundle By Name(cluster=w478, "Data"=w449) -> (w475:T9)
          n228 = for {
            tunnel: w449 -> [w483] mode=indexing
            tunnel: w448 -> [w481]
            tunnel: [w479] -> w447 mode=indexing
            n229 = Unbundle By Name(w483) -> ("Y"=w480:dbl)
            n230 = Subtract(x=w480, y=w481) -> (x-y=w482:dbl)
            n231 = Bundle By Name(cluster=w483, "Y"=w482) -> (w479:cluster{"X":dbl, "Y":dbl})
          }
          n232 = Bundle By Name(cluster=w460, "Maximum"=w461) -> (w456:T4)
          n233 = Replace Array Subset(array=w476, new element=w475, index=w453) -> (w474:T10)
          n234 = Less?(x=w458, y=w457) -> (x < y?=w459:bool)
          n235 = local read "Auto range"() -> (w450:bool)
          n236 = Bundle(w447) -> (w471:cluster{cluster{"X":dbl, "Y":dbl}[]})  [unwired: 1 in]
          n237 = Select(t=w458, s=w459, f=w457) -> (s? t:f=w455:dbl)
          n238 = Bundle By Name(cluster=w456, "Minimum"=w455) -> (w452:T4)
          n239 = case shown="True" w450 {
            tunnel: w454 -> [w484 w488]
            tunnel: w453 -> [_ w487]
            tunnel: w452 -> [_ w486]
            tunnel: [w484 w485] -> w451
            frame False {
            }
            frame True {
              n240 = Replace Array Subset(array=w488, new element=w486, index=w487) -> (w485:T1)
            }
          }
        }
        "Ranges" <- w432
      }
      frame True {
        n241 = local read "Instantaeneous data"() -> (w509:T2)
        n242 = local read "Time span (ms)"() -> (w497:dbl)
        n243 = Subtract(x=w497, y=w496) -> (x-y=w494:dbl)
        n244 = Subtract(x=w496, y=w497) -> (x-y=w493:dbl)
        n245 = Subtract(x=w493, y=0.0) -> (x-y=w492:dbl)
        n246 = Add(x=w502, y=w494) -> (x+y=w495:dbl)
        n247 = Add(x=w492, y=w497) -> (x+y=w498:dbl)
        n248 = Add(x=w501, y=w498) -> (x+y=w499:dbl)
        n249 = Add(x=w495, y=w498) -> (x+y=w500:dbl)
        n250 = Increment(x=w504) -> (x+1=w503:i32)
        n251 = for {
          shift-right: [w526] -> w508
          shift-left: w510 -> [w533]
          tunnel: w509 -> [w532] mode=indexing
          shift-right: [w529] -> w507
          shift-left: w506 -> [w529]
          tunnel: [w528] -> w505 mode=indexing
          tunnel: w500 -> [w521]
          tunnel: w499 -> [w520]
          shift-right: [w514] -> w489
          shift-left: w490 -> [w517]
          i -> [w516]
          n252 = Unbundle By Name(w532) -> ("Data"=w519:cluster{"X":dbl, "Y":dbl})
          n253 = Index Array(array=w533, index=w516) -> (element=w531:T9)
          n254 = Unbundle By Name(w519) -> ("X"=w527:dbl)
          n255 = Unbundle By Name(w519) -> ("Y"=w518:dbl)
          n256 = Build Array(w519) -> (w524:cluster{"X":dbl, "Y":dbl}[])
          n257 = In Range and Coerce(upper limit=w521, x=w527, lower limit=w520) -> (In Range?=w525:bool)  [unwired: 1 out]
          n258 = Select(t=w524, s=w525, f=cluster{"X":dbl, "Y":dbl}[] []) -> (s? t:f=w523:cluster{"X":dbl, "Y":dbl}[])
          n259 = Bundle By Name(cluster=T4 {"Maximum"=-1000000000.0, "Minimum"=1000000000.0, "Offset"=0.0}, "Maximum"=w518, "Minimum"=w518) -> (w515:T4)
          n260 = local read "Auto range"() -> (w513:bool)
          n261 = Bundle By Name(cluster=w531, "Data"=w523) -> (w530:T9)
          n262 = Bundle("f"=w523) -> (w528:cluster{"f":cluster{"X":dbl, "Y":dbl}[]})  [unwired: 1 in]
          n263 = Replace Array Subset(array=w533, new element=w530, index=w516) -> (w526:T10)
          n264 = case shown="True" w513 {
            tunnel: w517 -> [w534 w538]
            tunnel: w516 -> [_ w537]
            tunnel: w515 -> [_ w536]
            tunnel: [w534 w535] -> w514
            frame False {
            }
            frame True {
              n265 = Replace Array Subset(array=w538, new element=w536, index=w537) -> (w535:T1)
            }
          }
        }
        n266 = Tick Count (ms)() -> (millisecond timer value=w511:u32)
      }
    }
    n267 = local read "Channel 1 parameter"() -> (w404:string)
    n268 = local read "Channel 2 parameter"() -> (w403:string)
    n269 = local read "Channel 3 parameter"() -> (w402:string)
    n270 = local read "Channel 4 parameter"() -> (w401:string)
    n271 = local read "Channel 5 parameter"() -> (w400:string)
    n272 = local read "Channel 6 parameter"() -> (w399:string)
    n273 = local read "Channel 7 parameter"() -> (w398:string)
    n274 = local read "Channel 8 parameter"() -> (w397:string)
    n275 = local read "Channel 1 enable"() -> (w396:bool)
    n276 = local read "Channel 2 enable"() -> (w395:bool)
    n277 = local read "Channel 3 enable"() -> (w394:bool)
    n278 = local read "Channel 4 enable"() -> (w393:bool)
    n279 = local read "Channel 5 enable"() -> (w392:bool)
    n280 = local read "Channel 6 enable"() -> (w391:bool)
    n281 = local read "Channel 7 enable"() -> (w390:bool)
    n282 = local read "Channel 8 enable"() -> (w389:bool)
    n283 = Build Array(w404, w403, w402, w401, w400, w399, w398, w397) -> (w387:string[])
    n284 = Build Array(w396, w395, w394, w393, w392, w391, w390, w389) -> (w388:bool[])
    n285 = for {
      tunnel: w384 -> [w422] mode=indexing
      tunnel: [w421] -> w383 mode=indexing
      n286 = Unbundle By Name(w422) -> ("name"=w421:string)
    }
    n287 = for {
      tunnel: w388 -> [w428] mode=indexing
      tunnel: w387 -> [w429] mode=indexing
      tunnel: [w429] -> w372 mode=indexing if=w428
    }
    "Active Plot Names" <- w372
    n288 = for {
      tunnel: w372 -> [w424] mode=indexing
      tunnel: w386 -> [w427]
      tunnel: [w425] -> w385 mode=indexing
      tunnel: w383 -> [w423]
      n289 = Search 1D Array(1D array=w423, element=w424) -> (index of element=w426:i32)  [unwired: 1 in]
      n290 = Index Array(array=w427, index=w426) -> (element=w425:cluster{"f":cluster{"X":dbl, "Y":dbl}[]})
    }
    n291 = control-ref of="Live Plot"() -> (w405:refnum<vi>)
    n292 = property class="XYGraph (strict)"(reference=w405, error in=w406, "XScale.Minimum"=w379, "XScale.Maximum"=w382, "Value"=w385) -> (error out=w376:errorcluster)  [unwired: 1 out]
    n293 = local read "Stop Application"() -> (w415:bool)
    n294 = case shown="True" w373 {
      tunnel: w376 -> [w416 w420]
      tunnel: [w416 w419] -> w375
      tunnel: w374 -> [_ w417]
      frame False {
      }
      frame True {
        n295 = Generate User Event(user event=w417, event data cluster=TRUE, error in=w420) -> (error out=w419:errorcluster)  [unwired: 1 in, 1 out]
      }
    }
  }
  n296 = while {
    tunnel: w4 -> [w544]
    tunnel: [w540] -> w3
    shift-right: ["SYNC"] -> _
    shift-left: FALSE -> [w543]
    stop <- w545 stop-if-true
    n297 = Not(x=w543) -> (.not. x?=w542:bool)
    n298 = And(x=w542, y="SYNC") -> (x .and. y?=w541:bool)
    n299 = case shown="True" w541 {
      tunnel: w544 -> [w546 w553]
      tunnel: [w546 w547] -> w540
      frame False {
      }
      frame True {
        n300 = call "SDPC - Pause Transfer.vi"("error in (no error)"=w553, "Pause transfer"=TRUE) -> ("error out"=w551:errorcluster)  [unwired: 2 in, 1 out]
        n301 = local read "COM Port"() -> (w550:refnum<visa-resource-name>)
        n302 = call "SDCP Request Start.vi"("error in (no error)"=w551, "COM Port"=w550) -> ("error out"=w549:errorcluster)  [unwired: 1 out]
        n303 = call "SDPC - Pause Transfer.vi"("error in (no error)"=w549, "Pause transfer"=FALSE) -> ("error out"=w547:errorcluster)  [unwired: 2 in, 1 out]
      }
    }
    n304 = local read "Stop Application"() -> (w545:bool)
  }
  n305 = while {
    tunnel: w64 -> [w556]
    stop <- w554 stop-if-true
    n306 = Tick Count (ms)() -> (millisecond timer value=w557:u32)
    n307 = Subtract(x=w557, y=w556) -> (x-y=→"Time (ms)":u32)
    n308 = local read "Stop Application"() -> (w554:bool)
  }
  n309 = while {
    shift-right: [w565] -> _
    shift-left: w35 -> [w571]
    tunnel: w4 -> [w572]
    tunnel: [w564] -> w34
    stop <- w568 stop-if-true
    # "Instantaeneous plot data acquisition"
    n310 = call "SDPC - Pause Transfer.vi"("RD/nWR"=TRUE) -> ("Transfer paused"=w561:bool)  [unwired: 3 in, 1 out]
    n311 = Get Queue Status(queue=w571, error in (no error)=w572) -> (queue out=w566:refnum<queue>, error out=w567:errorcluster, # elements in queue=w563:i32)  [unwired: 1 in, 5 out]
    n312 = Not(x=w561) -> (.not. x?=w560:bool)
    n313 = Not Equal To 0?(x=w563) -> (x != 0?=w559:bool)
    n314 = And(x=w559, y=w560) -> (x .and. y?=w558:bool)
    n315 = case shown="True" w558 {
      tunnel: w567 -> [w573 w581]
      tunnel: w566 -> [w574 w580]
      tunnel: [w574 w579] -> w565
      tunnel: [w573 w576] -> w564
      frame False {
      }
      frame True {
        n316 = Dequeue Element(queue=w580, error in (no error)=w581) -> (queue out=w579:refnum<queue>, element=w577:T6, error out=w578:errorcluster)  [unwired: 1 in, 1 out]
        n317 = call "SDCP SMF Transmitter and Receiver - Live Plot - Obtain Instantaeneous Data Points.vi"("Raw frame"=w577, "error in (no error)"=w578) -> ("Instantaeneous data"=w575:T2, "error out"=w576:errorcluster)  [unwired: 4 in]
        n318 = local write "Instantaeneous data"(w575) -> ()
      }
    }
    n319 = Equal To 0?(x=w563) -> (x = 0?=w570:bool)
    n320 = local read "Stop Application"() -> (w569:bool)
    n321 = And(x=w569, y=w570) -> (x .and. y?=w568:bool)
  }
  n322 = call "SDCP SMF Transmitter and Receiver - Live Plot - Logger Loop.vi"("error in (no error)"=w4, "log queue"=w7) -> ("error out"=w8:errorcluster)  [unwired: 2 in, 1 out]
  n323 = Merge Errors(w34, w42, w8, w65, w3) -> (w37:errorcluster)
  n324 = Build Array(w41, w40, w39) -> (w38:refnum<queue>[])
  n325 = for {
    tunnel: w38 -> [w585] mode=indexing
    tunnel: w37 -> [w586]
    tunnel: [w582] -> w36
    n326 = Flush Queue(queue=w585, error in (no error)=w586) -> (queue out=w583:refnum<queue>, error out=w584:errorcluster)  [unwired: 1 out]
    n327 = Release Queue(queue=w583, error in (no error)=w584) -> (error out=w582:errorcluster)  [unwired: 1 in, 2 out]
  }
  n328 = call "SDCP - Serial Port Control.vi"("Command"=SDCP_-_Serial_Port_Control_-_Commands."Close", "error in (no error)"=w36) -> ("error out"=w67:errorcluster)  [unwired: 6 in, 3 out]
  n329 = disable-structure shown="Enabled" {
    disable-tunnel: w67 -> [w589 w590]
    disable-tunnel: enum16{"Initialize", "Acquire", "Save"}."Save" ("Command") -> [w588 _]
    disable-tunnel: [w587 w590] -> w59
    frame Disabled {
      n330 = call "SDCP SMF Receiver andTransmitter - Live Plot - Log File FGV.vi"("error in (no error)"=w589, "Command"=w588) -> ("error out"=w587:errorcluster)  [unwired: 5 in]
    }
    frame Enabled {
    }
  }
  n331 = disable-structure shown="Enabled" {
    disable-tunnel: w59 -> [w592 _]
    disable-tunnel: enum16{"Initialize", "Acquire", "Save"}."Save" ("Command") -> [w591 _]
    frame Disabled {
      n332 = call "SDCP SMF Receiver and Transmitter - Live Plot - Obtain Data Points.vi"("error in (no error)"=w592, "Command"=w591) -> ()  [unwired: 5 in, 1 out]
    }
    frame Enabled {
    }
  }
  "Live Plot" <- T3 [] ("Live Plot")
